vi "Create Basic Data Item.vi"(11 "Content":string) -> (3 "New Data Item":refnum<class "Data Item.lvclass">)   [LabVIEW 2023, in "VILab.lvlib" / "Data Item.lvclass"]
uses:
  Data Item.lvclass
  Data Item.lvclass/Data Item.ctl
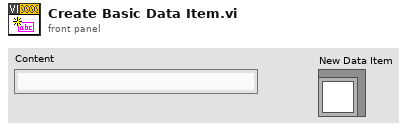
[diagram p1: front panel]
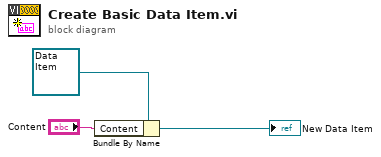
[diagram p0: block diagram]
diagram:
  n1 = Bundle By Name(cluster=refnum<class "Data Item.lvclass"> refnum ("VILab.lvlib:Data Item.lvclass"), "Content"="Content") -> (→"New Data Item":refnum<class "Data Item.lvclass">)
